vi "session.vi"() -> ()   [LabVIEW 2024]
panel:
  in  "Session":string
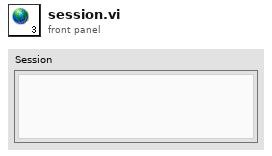
[diagram p1: front panel]
diagram:
